vi "DominicLastauskasLab02.vi"() -> ()   [LabVIEW 2024]
panel:
  out "Tank":dbl(slide) scale=-40000.0..40000.0
  out "Sensor Volts":dbl
  out "SCC Volts":dbl format="%.3f"
  out "Numeric":i32 format="%04x"
  in  "millisecond timer value":u32
  in  "stop":bool
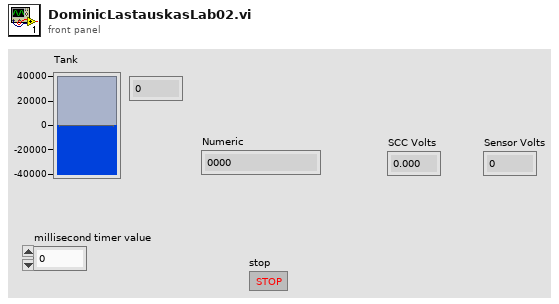
[diagram p1: front panel]
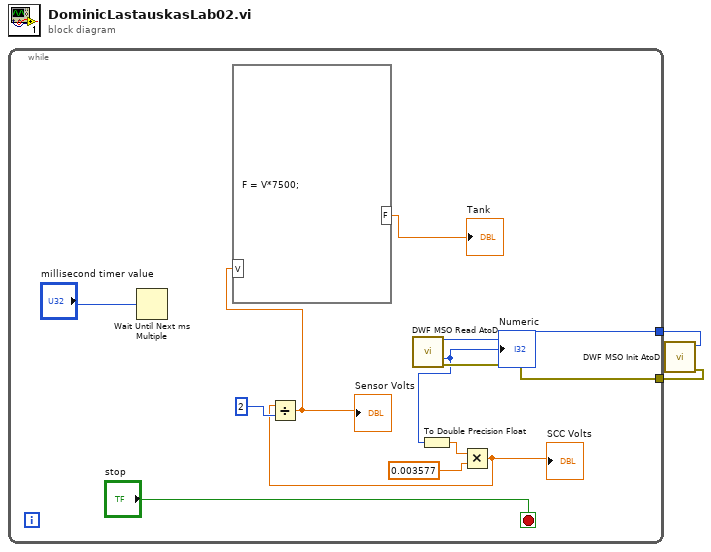
[diagram p0: block diagram]
diagram:
  n1 = call "DWF MSO Init AtoD.vi"() -> ("Error Out"=w1:errorcluster, "Instrument Handle Out"=w2:u32)  [unwired: 10 in]
  n2 = while {
    tunnel: w2 -> [w11]
    tunnel: w1 -> [w10]
    stop <- "stop" stop-if-true
    n3 = Wait Until Next ms Multiple(millisecond multiple="millisecond timer value") -> ()  [unwired: 1 out]
    n4 = call "DWF MSO Read AtoD.vi"("Instrument Handle In AtoD"=w11, "Error In"=w10) -> ("AtoD"=w9:i16)  [unwired: 12 in, 1 out]
    "Numeric" <- w9
    n5 = To Double Precision Float(number=w9) -> (double precision float=w8:dbl)
    n6 = Multiply(x=w8, y=0.003577) -> (x*y=w5:dbl)
    "SCC Volts" <- w5
    n7 = Divide(x=w5, y=2) -> (x/y=w4:dbl)
    "Sensor Volts" <- w4
    n8 = formula code="F = V*7500;"("V"=w4) -> ("F"=→"Tank":dbl)
  }
